vi "Fix_angle.vi"(3 "±180 -> 0-360?":bool, 4 "Angle IN":dbl) -> (1 "Angle OUT":dbl)   [LabVIEW 2019]
panel:
  # "Converti un angle entre 0° et 360° à la notation ±180°"
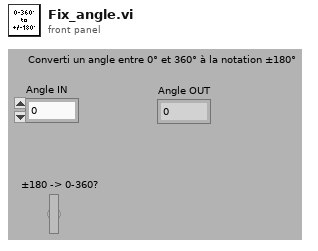
[diagram p1: front panel]
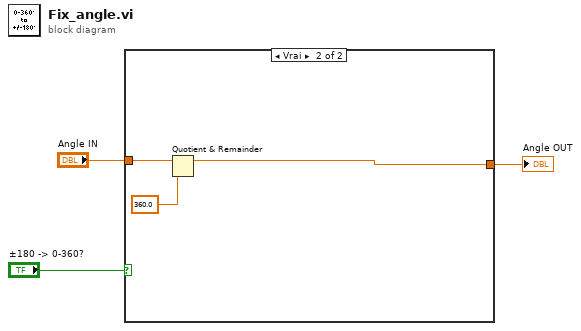
[diagram p0: block diagram]
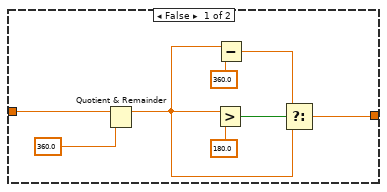
[diagram p2: hidden frame]
diagram:
  n1 = case shown="Vrai" "±180 -> 0-360?" {
    tunnel: [w7 w12] -> w3
    tunnel: "Angle IN" -> [w6 w14]
    frame False {
      n2 = Quotient & Remainder(x=w6, y=360.0) -> (x-y*floor(x/y)=w4:dbl)  [unwired: 1 out]
      n3 = Greater?(x=w4, y=180.0) -> (0:w11:bool)
      n4 = Subtract(x=w4, y=360.0) -> (x-y=w8:dbl)
      n5 = Select(t=w8, s=w11, f=w4) -> (s? t:f=w7:dbl)
    }
    frame True {
      n6 = Quotient & Remainder(x=w14, y=360.0) -> (x-y*floor(x/y)=w12:dbl)  [unwired: 1 out]
    }
  }
  "Angle OUT" <- w3
